vi "LinearFilter_HighPassBW2.vi"(9 "SamplePeriod":dbl format="%13.5p", 11 "TimeConstant":dbl format="%13.5p") -> (3 "LINEAR_FILTER":T1 {"Outputs" format="%13.5g"; "Inputs" format="%13.5g"; "OutputGains" format="%13.5g"; "InputGains" format="%13.5g"})   [LabVIEW 2019, in "Trajectory_Library.lvlib"]
doc: "Creates a 2nd order Butterworth high pass filter.\n\nA 2nd order filter provides more filtering, however it also has a larger phase shift (time delay).\n\nMore information on this type of filter can be found at:\n\n https://en.wikipedia.org/wiki/Butterworth_filter\n\nInputs: \n - timeConstant - The discrete-time time constant in seconds.\n - samplePeriod - The period in seconds between samples taken by the user.\n\nOutputs:\n - Linearfilter - Created datat structure"
uses:
  Trajectory_Library.lvlib
  TypeDef/LINEAR_FILTER.ctl
  <vilib>/Rock Robotics/SystemInterfaces/NetworkCommunication/NetComm_UsageReport_report.vi
  Globals/Util_LibraryGlobals.vi
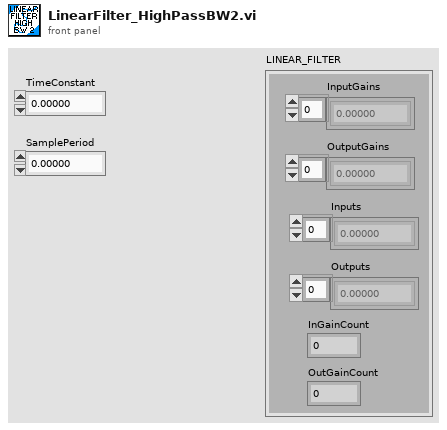
[diagram p1: front panel]
types:
  T1 = typedef "Trajectory_Library.lvlib/LINEAR_FILTER.ctl" = cluster{"InputGains":dbl[], "OutputGains":dbl[], "Inputs":dbl[], "Outputs":dbl[], "InGainCount":i32, "OutGainCount":i32}
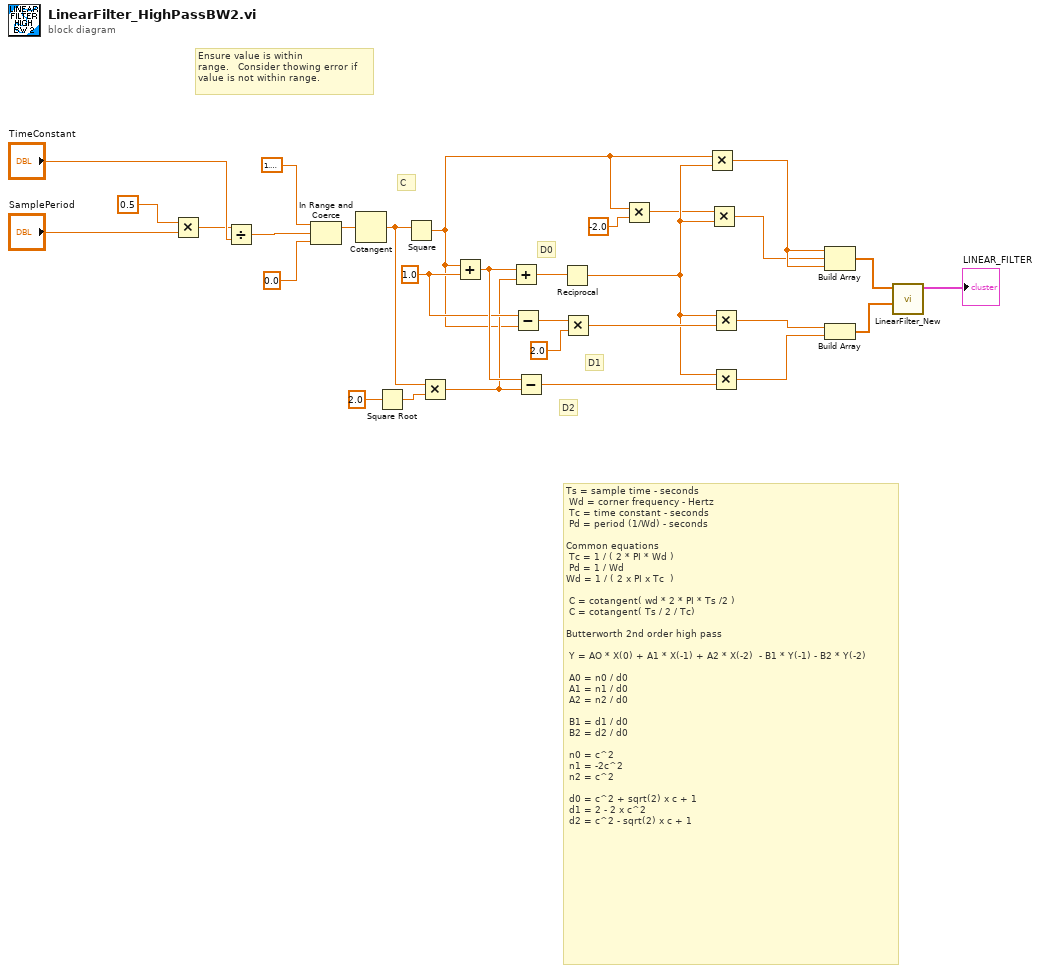
[diagram p0: block diagram]
diagram:
  w17 = 1.0 ("y")
  # "Ensure value is within\nrange.   Consider thowing error if\nvalue is not within range."
  # "D1"
  # "D2"
  # "D0"
  # "Ts = sample time - seconds\n\tWd = corner frequency - Hertz\n\tTc = time constant - seconds\n\tPd = period (1/Wd) - seconds\n\nCommon equations\n\tTc = 1 / ( 2 * PI * Wd )\n\tPd = 1 / Wd\nWd = 1 / ( 2 x PI x Tc  )\n\t\n\tC = cotangent( wd * 2 * PI * Ts /2 )\n C = cotangent( Ts / 2 / Tc)\n\nButterworth 2nd order high pass\n\n\tY = AO * X(0) + A1 * X(-1) + A2 * X(-2)  - B1 * Y(-1) - B2 * Y(-2) \n\n\tA0 = n0 / d0\n\tA1 = n1 / d0\n\tA2 = n2 / d0\n\n\tB1 = d1 / d0\n\tB2 = d2 / d0\n\n\tn0 = c^2\n\tn1 = -2c^2\n n2 = c^2\n\n\td0 = c^2 + sqrt(2) x c + 1\n\td1 = 2 - 2 x c^2\n\td2 = c^2 - sqrt(2) x c + 1"
  # "C"
  n1 = Multiply(x=0.5, y="SamplePeriod") -> (x*y=w26:dbl)
  n2 = Divide(x=w26, y="TimeConstant") -> (x/y=w21:dbl)
  n3 = In Range and Coerce(upper limit=1.5707963267948966, x=w21, lower limit=0.0) -> (coerced(x)=w20:dbl)  [unwired: 1 out]
  n4 = Cotangent(1:w20) -> (0:w7:dbl)
  n5 = Square Root(x=2.0) -> (sqrt(x)=w9:dbl)
  n6 = Square(x=w7) -> (x^2=w5:dbl)
  n7 = Multiply(x=w7, y=w9) -> (x*y=w8:dbl)
  n8 = Add(x=w5, y=w17) -> (x+y=w18:dbl)
  n9 = Add(x=w18, y=w8) -> (x+y=w14:dbl)
  n10 = Subtract(x=w17, y=w5) -> (x-y=w15:dbl)
  n11 = Subtract(x=w18, y=w8) -> (x-y=w13:dbl)
  n12 = Reciprocal(x=w14) -> (1/x=w3:dbl)
  n13 = Multiply(x=w15, y=2.0) -> (x*y=w12:dbl)
  n14 = Multiply(x=w5, y=-2.0) -> (x*y=w2:dbl)
  n15 = Multiply(x=w5, y=w3) -> (x*y=w6:dbl)
  n16 = Multiply(x=w2, y=w3) -> (x*y=w1:dbl)
  n17 = Multiply(x=w3, y=w12) -> (x*y=w10:dbl)
  n18 = Multiply(x=w3, y=w13) -> (x*y=w11:dbl)
  n19 = Build Array(w6, w1, w6) -> (w30:dbl[])
  n20 = Build Array(w10, w11) -> (w28:dbl[])
  n21 = call "LinearFilter_New.vi"("OutputGains"=w28, "InputGains"=w30) -> ("LINEAR_FILTER"=→"LINEAR_FILTER":T1)  [unwired: 9 in]
